vi "Z6_Beamline.panel.vi"(0 "object ref":refnum<vi>, 5 "error in (no error)":errorcluster) -> (19 "error out":errorcluster)   [LabVIEW 2014, in "Z6_Beamline.lvlib"]
doc: "By this VI a hardware switch can be monitored and switched. \n\nThe indicators \"FALSE\", \"TRUE\" and \"SWITCH STATE\" show the value of the Beckhoff-Tag: blue indicates bad tag status reference problems, darkgreen false and lightgreen true. If everything is working fine, \"FALSE\" and \"SWITCH STATE\" should show the same value, while \"TRUE\" has the opposite value. The caption of the sensors for \"FALSE\" and \"TRUE\" are taken out of the database. In case of only one or no sensor these GUI elements are not shown at all.\n\nThe oval button switches. It should be in the same state as the \"SWITCH STATE\" indicator. \n\n\"Delete Instance\" disconnects and removes the instance from the PCS.\n\n\nLicense Agreement for this software:\n\nCopyright (C)\nGesellschaft für Schwerionenforschung, GSI\nPlanckstr. 1\n64291 Darmstadt\nGermany\n\nContact: D.Beck@gsi.de \n\nThis program is free software; you can redistribute it and/or modify it under the terms of the GNU General Public License as published by the Free Software Foundation; either version 2 of the license, or (at your option) any later version.\n\nThis program is distributed in the hope that it will be useful, but WITHOUT ANYW ARRANTY; without even the implied warranty of MERCHANTABILITY or FITNESS FOR A PARTICULAR PURPOSE. See the GNU General License for more details (http://www.gnu.org).\n\nGesellschaft für Schwerionenforschung, GSI\nPlanckstr. 1, 64291 Darmstadt, Germany\nFor all questions and ideas contact: M.Richter@gsi.de, H.Brand@gsi.de or D.Beck@gsi.de.\nLast update: 18-DEC-2002"
uses:
  Z6_Beamline.lvlib
  PH_Common/Picture/PH_Picture.GUI Element 36x36.ctl
  PH_Common/Picture/PH_Picture.GUI Element 24x36.ctl
  PH_Common/Picture/PH_Picture.GUI Element.ctl
  Z6_Beamline.Switch Instances.ctl
  Z6_Beamline.Black Box Instances.ctl
  PH_SystemInformation/PH_SystemInformation.GUI Refs.ctl
  PH_BL-Master/PH_BL-Master.GUI Refs.ctl
  Z6_Beamline.Subsystem ok GUI Refs.ctl
  Z6_Beamline.GUI Refs.ctl
  PH_Common/PH_Common.lvlib
  PH_Switch/PH_Switch.lvlib
  PH_BlackBox/PH_BlackBox.lvlib
  PH_BL-Master/PH_BL-Master.lvlib
  PH_Class/PH_Class.lvlib
  PH_SystemInformation/PH_SystemInformation.lvlib
panel:
  in  "Z6 Black Box Instances":T1="Z6_ST_Attenuator_1_BB"
  in  "Z6 Switch Instances":T2="Shutter_Exp4"
  out "Exp 3":u32(colorbox)
  out "Exp 2":u32(colorbox)
  out "Exp 1":u32(colorbox)
  out "Emergency Off":u32(colorbox)
  in  "Remote Desktop Connection":bool
  out "PHELIX_Timing_Mode":enum32{"10 Hz", "0.5 Hz", "Shot"}(radio) caption="Modeselector"
  in  "PCS System Indicator":bool caption="PCS"
  in  "CoG":bool
  in  "Calibrator":bool
  in  "Image Statistician":bool
  in  "Z6 Main":bool
  out "Exp 4 (Z6)":u32(colorbox)
  in  "Tab Control":T3(tab)
  in  "PA_CH1_BB":T4 caption="CH"
  in  "ns_WP_RR_6PWpGUI":T5 caption="Waveplate ns Frontend"
  in  "YLF_WP_6PWpGUI":T5 caption="Waveplate YLF"
  in  "fs_WP_Exit_6PWpGUI":T5 caption="Waveplate fs Frontend"
  in  "Hop 3":bool
  out "Frontends ok":bool caption="ok"
  in  "MA_MM8_6PGUI":T6
  in  "MA_MM9_6PGUI":T6
  out "MA_VacuumControl::MA_VacuumControl_Z6 Telescope BL Prepressure":dbl=2000.0 caption="mbar" format="%#_2e"
  in  "BL-Z6-CH10":T4
  out "BL NT 2":u32(colorbox)
  in  "BL-Z6-CH9":T4
  in  "BL-Z6-Beamdump":bool=TRUE
  in  "Hop 4":bool
  in  "Z6_SHG_TIP-TILT_6PGUI":T6
  in  "Z6_SHG_ROT_6PGUI":T6
  out "MA_VacuumControl::MA_VacuumControl_Z6 Telescope BL":dbl=2000.0 caption="mbar" format="%#_2e"
  out "BL NT 3":u32(colorbox)
  in  "Z6_MM10_6PGUI":T6
  in  "Hop 1":bool
  out "Shutter_Exp4":bool=TRUE
  in  "\"D:\\PCS\\Remote Access\\Z6-Northtower.rdp\"":bool caption="OK Button"
  out "Northtower ok":bool caption="ok"
  in  "\"D:\\PCS\\Remote Access\\Z6-Southtower.rdp\"":bool caption="OK Button"
  out "Southtower ok":bool caption="ok"
  in  "Z6_ST_Attenuator_1_BB":bool=TRUE
  in  "Z6_ST_Attenuator_2_BB":T5 caption="BB 2"
  in  "Z6_green_Alignment_Powermeter":bool=TRUE
  in  "BL-Z6-CH11":T4
  in  "Z6_ST_WP_6PWpGUI":T5 caption="Waveplate"
  in  "Hop 5":bool
  in  "Z6_ST_NF_green_Cam":bool=TRUE caption="PA NF Exit Cam"
  in  "Z6_green_Powermeter":bool=TRUE
  out "BL ST 10":u32(colorbox)
  out "BL ST 9":u32(colorbox)
  out "BL ST 8":u32(colorbox)
  out "BL ST 7":u32(colorbox)
  in  "Z6_IR_Powermeter":bool=TRUE
  out "BL ST 6":u32(colorbox)
  in  "Z6_ST_NF_IR_Cam":bool=TRUE caption="PA FF Exit Cam"
  out "BL ST 5":u32(colorbox)
  out "BL ST 4":u32(colorbox)
  out "BL ST 3":u32(colorbox)
  out "BL ST 1":u32(colorbox)
  in  "Hop 2":bool
  out "BL ST 2":u32(colorbox)
  in  "Z6_MM11_6PGUI":T6
  in  "Z6_ST_Flip_Cam_BB":T6
  in  "Z6_ST_Flip_PD_BB":T6
  in  "\"D:\\PCS\\Remote Access\\Z6-Compressor.rdp\"":bool caption="OK Button"
  in  "Z6_ST_COS_Sensitivity_Switch_BB":bool=TRUE
  in  "Z6_ST_COS_WP_6PWpGUI":T5 caption="Waveplate"
  in  "Z6_ST_COS_Filt_1_BB":T5 caption="Filt 1"
  in  "Z6_ST_COS_Filt_2_BB":bool=TRUE
  in  "Z6_COS_Powermeter":bool=TRUE
  out "BL 100TW COS 6":u32(colorbox)
  out "BL 100TW COS 5":u32(colorbox)
  in  "Z6_Compressor-SSAC":bool=TRUE
  in  "Z6_COS_SSAC_Cam":bool=TRUE caption="PA NF Exit Cam"
  in  "Z6_COS_NF_ImageOperator":bool=TRUE
  in  "Z6_COS_NF_Cam":bool=TRUE caption="PA NF Exit Cam"
  in  "Z6_COS_FF_Cam":bool=TRUE caption="PA FF Exit Cam"
  in  "Hop 6":bool
  out "100TW COS ok":bool caption="ok"
  out "Ready for Shot":bool
  out "MainAmp enabled":u32(colorbox)
  out "Laser enabled":u32(colorbox)
  out "PreAmp enabled":u32(colorbox)
  in  "Minimize":bool
  in  "Delete":bool
  out "loop counter":i32
  # "Z6-CS"
  # "3.40"
  # "2"
  # "1"
  # "GREEN"
  # "IR"
  # "1"
  # "2"
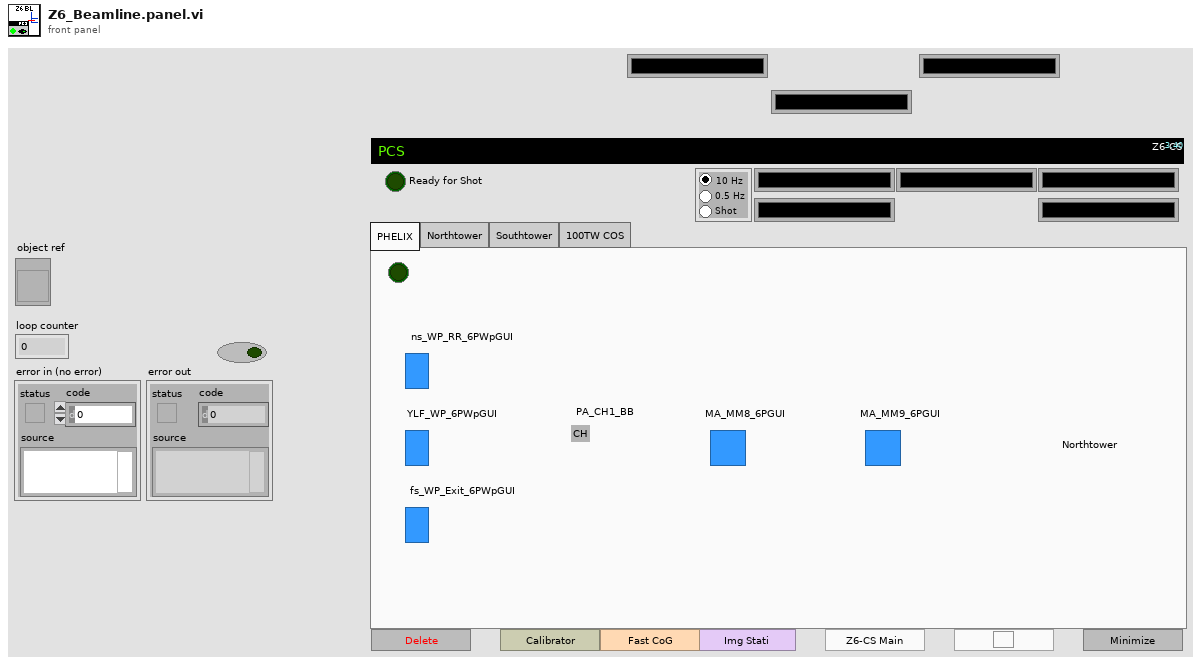
[diagram p1: front panel]
types:
  T1 = typedef "Z6_Beamline.lvlib/Z6_Beamline.Black Box Instances.ctl" = string
  T2 = typedef "Z6_Beamline.lvlib/Z6_Beamline.Switch Instances.ctl" = string
  T3 = enum32{"PHELIX", "Northtower", "Southtower", "100TW COS"}
  T4 = typedef "PH_Common.lvlib/PH_Picture.GUI Element.ctl" = picture
  T5 = typedef "PH_Common.lvlib/PH_Picture.GUI Element 24x36.ctl" = picture
  T6 = typedef "PH_Common.lvlib/PH_Picture.GUI Element 36x36.ctl" = picture
  T7 = typedef "Z6_Beamline.lvlib/Z6_Beamline.GUI Refs.ctl" = cluster{"BL NT":refnum<vi>[], "BL ST":refnum<vi>[], "BL 100 TW COS":refnum<vi>[], "Subs ok GUI Refs":T8}
  T8 = typedef "Z6_Beamline.lvlib/Z6_Beamline.Subsystem ok GUI Refs.ctl" = cluster{"Northtower ok":refnum<vi>, "Southtower ok":refnum<vi>, "Frontends ok":refnum<vi>, "100TW COS ok":refnum<vi>}
  T9 = typedef "PH_BL-Master.lvlib/PH_BL-Master.GUI Refs.ctl" = cluster{"Vac GUI Refs":refnum<vi>[], "O2 GUI Refs":refnum<vi>[], "Ready for Shot":refnum<vi>, "Boolean Condition Service Subscriber GUI Refs":refnum<vi>[], "Vision ID on same Node":string, "Picture Condition Service Subscriber GUI Refs":refnum<vi>[], "6P 4Q GUI Refs":refnum<vi>[], "Ref Switch GUI Instances":refnum<vi>, "Ref 6P Switch Instances":refnum<vi>, "Ref BB Instances":refnum<vi>, "Ref Switch Instances":refnum<vi>, "Ref Switch and 6P State Instances":refnum<vi>, "Boolean Status Service Subscriber GUI Refs":refnum<vi>[], "Picture Status Service Subscriber GUI Refs":refnum<vi>[], "Force Sensor Instances":refnum<vi>, "GUI Ref Delete":refnum<vi>}
  T10 = typedef "PH_SystemInformation.lvlib/PH_SystemInformation.GUI Refs.ctl" = cluster{"Laser":refnum<vi>, "PreAmp":refnum<vi>, "MainAmp":refnum<vi>, "Emergency Off":refnum<vi>, "Exp 1":refnum<vi>, "Exp 2":refnum<vi>, "Exp 3":refnum<vi>, "Exp 4":refnum<vi>, "Timing Mode GUI Ref":refnum<vi>}
  T11 = enum16{"PCS", "Laser", "Vision", "PP", "Special", "Beckhoff"}
  T12 = enum16{"None", "PCS Main", "Z6 Main", "PCS Beamline", "Z6 Beamline", "Image Statistician", "Powermeter Statistician", "SHS Anal Statistician", "Image Center of Gravity", "Image Calibrator", "SHS Analysis Calibrator", "Cam List", "Powermeterlist", "6P List", "BB List", "Switch List", "Sequence Watch"}
  T13 = typedef "PH_BL-Master.lvlib/PH_BL-Master.i attribute.ctl" = cluster{"Remote controlled":bool, "Boolean Condition Service Subscriber":refnum<vi>[], "Picture Condition Service Subscriber":refnum<vi>[], "R2S":cluster{"GUI Ref":refnum<vi>, "State":bool}, "Vacua":cluster{"GUI Ref":refnum<vi>, "Limit":dbl, "Curr Value":dbl, "in range":bool}[], "O2 Inspection":cluster{"GUI Ref":refnum<vi>, "Concentration":dbl, "State":T14}[], "Boolean Status Service Subscriber":cluster{"GUI Ref":refnum<vi>, "Status":T14, "no Link?":bool, "Status Subscriber Class":T15}[], "Picture Status Service Subscriber":cluster{"GUI Ref":refnum<vi>, "Status":T14, "no Link?":bool, "Status Subscriber Class":T15}[], "6P 4Q Service Subscriber":cluster{"GUI Ref":refnum<vi>, "Selector":T16, "no Link?":bool}[], "Index of latest 6P 4Q changing Instance":i32, "Index of latest Picture Status changing Instance":i32, "Index of latest Boolean Status changing Instance":i32, "Vision ID on same Node":string, "Start Phase over?":bool, "GUI Ref Delete":refnum<vi>}
  T14 = typedef "PH_StatusHandler.lvlib/PH_StatusHandler.Status.ctl" = i16
  T15 = typedef "PH_BL-Master.lvlib/PH_BL-Master.Status Subscriber Class.ctl" = enum16{"unknown", "Switch", "BB", "6P Switch", "Switch GUI", "Switch and 6P State", "Force Sensor"}
  T16 = typedef "PH_4_Pos_Selector.lvlib/PH_4_Pos_Selector.Position Selector.ctl" = u16
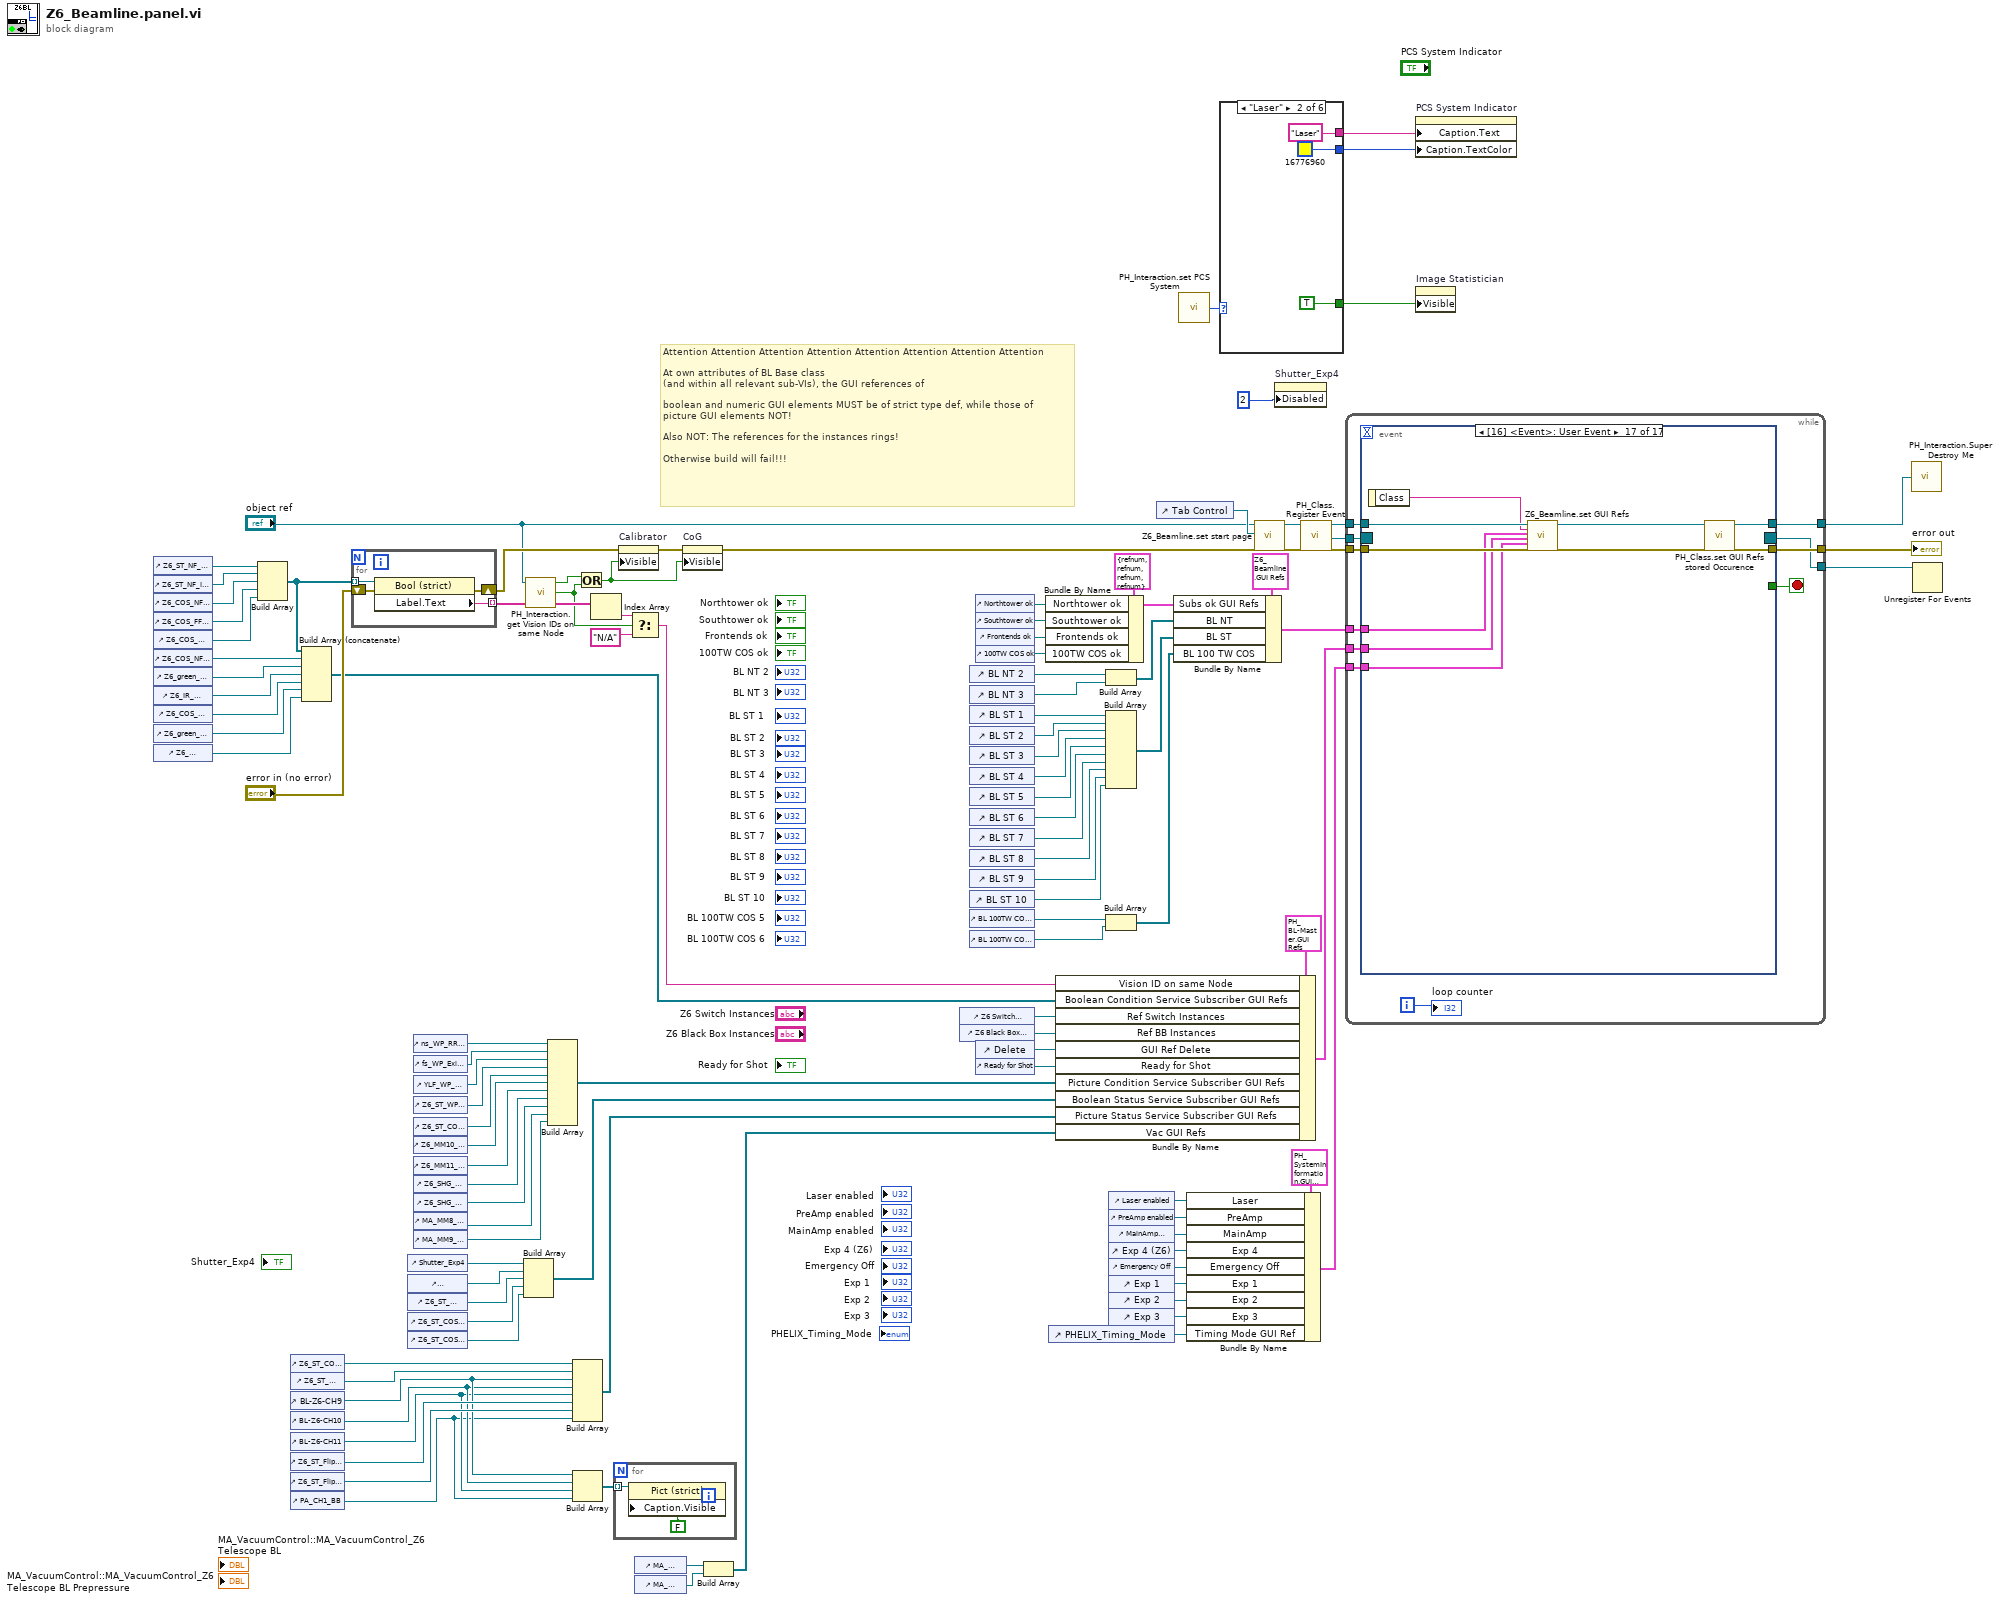
[diagram p0: block diagram]
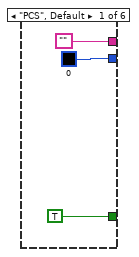
[diagram p2: hidden frame]
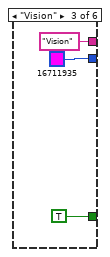
[diagram p3: hidden frame]
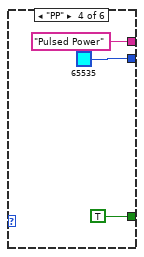
[diagram p4: hidden frame]
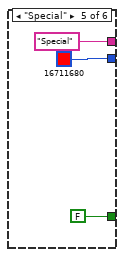
[diagram p5: hidden frame]
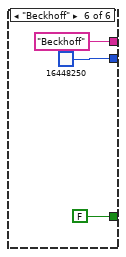
[diagram p6: hidden frame]
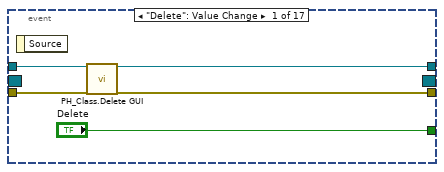
[diagram p7: hidden frame]
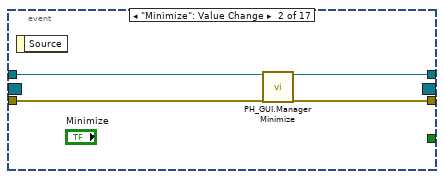
[diagram p8: hidden frame]
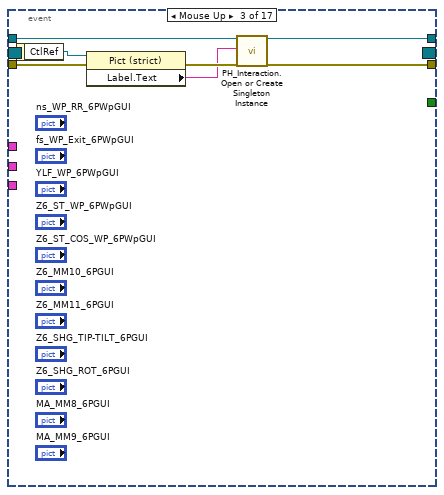
[diagram p9: hidden frame]
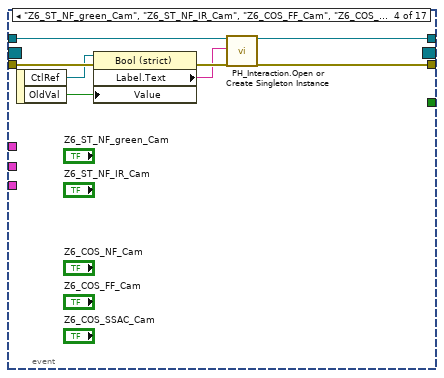
[diagram p10: hidden frame]
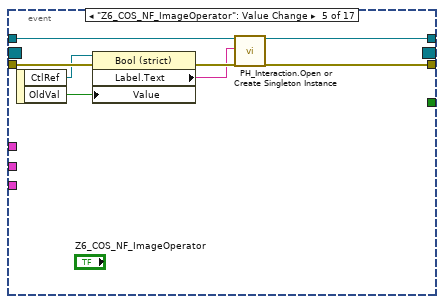
[diagram p11: hidden frame]
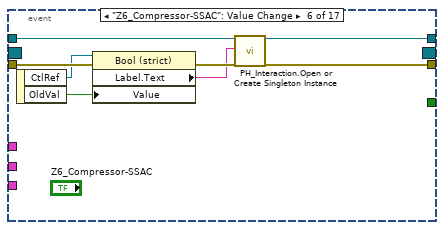
[diagram p12: hidden frame]
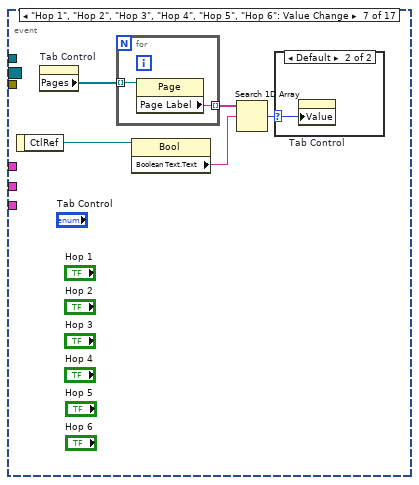
[diagram p13: hidden frame]
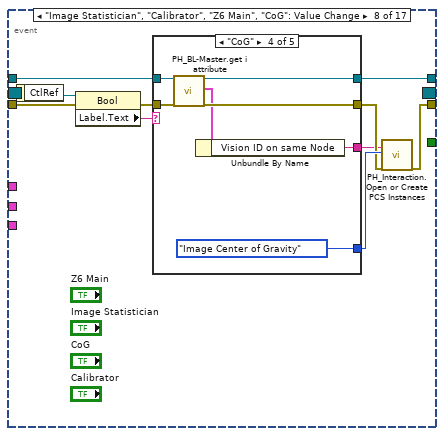
[diagram p15: hidden frame]
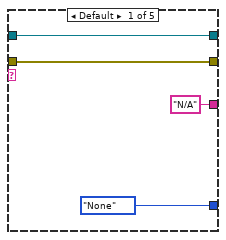
[diagram p16: hidden frame]
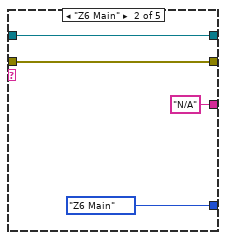
[diagram p17: hidden frame]
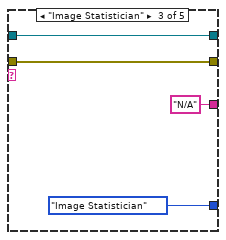
[diagram p18: hidden frame]
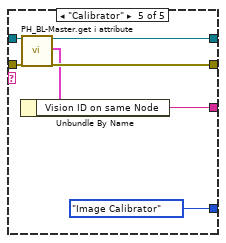
[diagram p19: hidden frame]
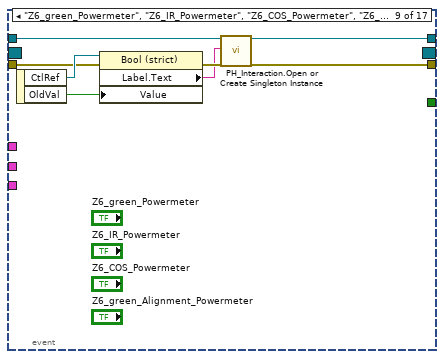
[diagram p20: hidden frame]
diagram:
  # "Attention Attention Attention Attention Attention Attention Attention Attention\n\nAt own attributes of BL Base class \n(and within all relevant sub-VIs), the GUI references of\n\nboolean and numeric GUI elements MUST be of strict type def, while those of\npicture GUI elements NOT!\n\nAlso NOT: The references for the instances rings!\n\nOtherwise build will fail!!!"
  n1 = control-ref of="Z6_ST_NF_green_Cam"() -> (w48:refnum<vi>)
  n2 = control-ref of="Z6_ST_NF_IR_Cam"() -> (w47:refnum<vi>)
  n3 = control-ref of="Z6_COS_NF_Cam"() -> (w46:refnum<vi>)
  n4 = control-ref of="Z6_COS_FF_Cam"() -> (w45:refnum<vi>)
  n5 = control-ref of="Z6_COS_SSAC_Cam"() -> (w44:refnum<vi>)
  n6 = control-ref of="Z6_COS_NF_ImageOperator"() -> (w67:refnum<vi>)
  n7 = control-ref of="Z6_green_Powermeter"() -> (w64:refnum<vi>)
  n8 = control-ref of="Z6_IR_Powermeter"() -> (w63:refnum<vi>)
  n9 = control-ref of="Z6_COS_Powermeter"() -> (w62:refnum<vi>)
  n10 = control-ref of="Z6_green_Alignment_Powermeter"() -> (w61:refnum<vi>)
  n11 = control-ref of="Z6_Compressor-SSAC"() -> (w60:refnum<vi>)
  n12 = Build Array(w48, w47, w46, w45, w44) -> (w43:refnum<vi>[])
  n13 = control-ref of="Z6_ST_COS_Filt_1_BB"() -> (w88:refnum<vi>)
  n14 = control-ref of="Z6_ST_Attenuator_2_BB"() -> (w87:refnum<vi>)
  n15 = control-ref of="BL-Z6-CH9"() -> (w75:refnum<vi>)
  n16 = control-ref of="BL-Z6-CH10"() -> (w74:refnum<vi>)
  n17 = control-ref of="BL-Z6-CH11"() -> (w73:refnum<vi>)
  n18 = control-ref of="Z6_ST_Flip_Cam_BB"() -> (w79:refnum<vi>)
  n19 = control-ref of="Z6_ST_Flip_PD_BB"() -> (w78:refnum<vi>)
  n20 = control-ref of="PA_CH1_BB"() -> (w56:refnum<vi>)
  n21 = Build Array (concatenate)(w43, w67, w64, w63, w62, w61, w60) -> (w2:refnum<vi>[])
  n22 = for {
    shift-right: [w115] -> w22
    shift-left: "error in (no error)" -> [w116]
    tunnel: [w114] -> w51 mode=indexing
    tunnel: w43 -> [w113] mode=indexing
    n23 = property class="Bool (strict)"(reference=w113, error in=w116) -> (error out=w115:errorcluster, "Label.Text"=w114:string)  [unwired: 1 out]
  }
  n24 = control-ref of="Shutter_Exp4"() -> (w66:refnum<vi>)
  n25 = control-ref of="BL-Z6-Beamdump"() -> (w65:refnum<vi>)
  n26 = control-ref of="Z6_ST_Attenuator_1_BB"() -> (w59:refnum<vi>)
  n27 = control-ref of="Z6_ST_COS_Sensitivity_Switch_BB"() -> (w58:refnum<vi>)
  n28 = control-ref of="Z6_ST_COS_Filt_2_BB"() -> (w57:refnum<vi>)
  n29 = control-ref of="ns_WP_RR_6PWpGUI"() -> (w86:refnum<vi>)
  n30 = control-ref of="fs_WP_Exit_6PWpGUI"() -> (w85:refnum<vi>)
  n31 = control-ref of="YLF_WP_6PWpGUI"() -> (w84:refnum<vi>)
  n32 = control-ref of="Z6_ST_WP_6PWpGUI"() -> (w83:refnum<vi>)
  n33 = control-ref of="Z6_ST_COS_WP_6PWpGUI"() -> (w82:refnum<vi>)
  n34 = control-ref of="Z6_MM10_6PGUI"() -> (w81:refnum<vi>)
  n35 = control-ref of="Z6_MM11_6PGUI"() -> (w80:refnum<vi>)
  n36 = control-ref of="Z6_SHG_ROT_6PGUI"() -> (w77:refnum<vi>)
  n37 = control-ref of="Z6_SHG_TIP-TILT_6PGUI"() -> (w76:refnum<vi>)
  n38 = control-ref of="MA_MM8_6PGUI"() -> (w39:refnum<vi>)
  n39 = control-ref of="MA_MM9_6PGUI"() -> (w38:refnum<vi>)
  n40 = Build Array(w66, w65, w59, w58, w57) -> (w25:refnum<vi>[])
  n41 = call "PH_Interaction.get Vision IDs on same Node.vi"("Cam Instances"=w51, "i ref in"="object ref") -> ("Vision System IDs"=w42:string[], "Vision Sytem IDs found"=w40:bool, "Cams instanciated on own system"=w41:bool)  [unwired: 1 in]
  n42 = Build Array(w86, w85, w84, w83, w82, w81, w80, w77, w76, w39, w38) -> (w26:refnum<vi>[])
  n43 = Build Array(w88, w87, w75, w74, w73, w79, w78, w56) -> (w24:refnum<vi>[])
  n44 = Build Array(w75, w74, w73, w56) -> (w72:refnum<vi>[])
  n45 = Or(x=w41, y=w40) -> (x .or. y?=w21:bool)
  n46 = Index Array(array=w42) -> (element=w50:string)  [unwired: 1 in]
  n47 = for {
    tunnel: w72 -> [w118] mode=indexing
    n48 = property class="Pict (strict)"(reference=w118, "Caption.Visible"=FALSE) -> ()  [unwired: 1 in, 2 out]
  }
  n49 = property on="Calibrator" class="Bool"(error in=w22, "Visible"=w21) -> (error out=w23:errorcluster)  [unwired: 1 in, 1 out]
  n50 = Select(t=w50, s=w40, f="N/A") -> (s? t:f=w3:string)
  n51 = control-ref of="MA_VacuumControl::MA_VacuumControl_Z6 Telescope BL"() -> (w107:refnum<vi>)
  n52 = control-ref of="MA_VacuumControl::MA_VacuumControl_Z6 Telescope BL Prepressure"() -> (w37:refnum<vi>)
  n53 = property on="CoG" class="Bool"(error in=w23, "Visible"=w21) -> (error out=w18:errorcluster)  [unwired: 1 in, 1 out]
  n54 = Build Array(w107, w37) -> (w1:refnum<vi>[])
  n55 = control-ref of="Z6 Switch Instances"() -> (w29:refnum<vi>)
  n56 = control-ref of="Z6 Black Box Instances"() -> (w28:refnum<vi>)
  n57 = control-ref of="BL NT 2"() -> (w111:refnum<vi>)
  n58 = control-ref of="BL NT 3"() -> (w110:refnum<vi>)
  n59 = control-ref of="BL ST 1"() -> (w106:refnum<vi>)
  n60 = control-ref of="BL ST 2"() -> (w105:refnum<vi>)
  n61 = control-ref of="BL ST 3"() -> (w96:refnum<vi>)
  n62 = control-ref of="BL ST 4"() -> (w95:refnum<vi>)
  n63 = control-ref of="BL ST 5"() -> (w94:refnum<vi>)
  n64 = control-ref of="BL ST 6"() -> (w93:refnum<vi>)
  n65 = control-ref of="BL ST 7"() -> (w92:refnum<vi>)
  n66 = control-ref of="BL ST 8"() -> (w91:refnum<vi>)
  n67 = control-ref of="BL ST 9"() -> (w90:refnum<vi>)
  n68 = control-ref of="BL ST 10"() -> (w89:refnum<vi>)
  n69 = control-ref of="BL 100TW COS 5"() -> (w103:refnum<vi>)
  n70 = control-ref of="BL 100TW COS 6"() -> (w102:refnum<vi>)
  n71 = control-ref of="Northtower ok"() -> (w11:refnum<vi>)
  n72 = control-ref of="Southtower ok"() -> (w10:refnum<vi>)
  n73 = control-ref of="Frontends ok"() -> (w9:refnum<vi>)
  n74 = control-ref of="100TW COS ok"() -> (w8:refnum<vi>)
  n75 = control-ref of="Delete"() -> (w6:refnum<vi>)
  n76 = control-ref of="Ready for Shot"() -> (w27:refnum<vi>)
  n77 = Bundle By Name(cluster=T8 {"Northtower ok"=refnum, "Southtower ok"=refnum, "Frontends ok"=refnum, "100TW COS ok"=refnum} ("Subs ok GUI Refs"), "Northtower ok"=w11, "Southtower ok"=w10, "Frontends ok"=w9, "100TW COS ok"=w8) -> (w12:T8)
  n78 = control-ref of="PHELIX_Timing_Mode"() -> (w36:refnum<vi>)
  n79 = Bundle By Name(cluster=T9 {"Vac GUI Refs"=[], "O2 GUI Refs"=[], "Ready for Shot"=refnum, "Boolean Condition Service Subscriber GUI Refs"=[], "Vision ID on same Node"="", "Picture Condition Service Subscriber GUI Refs"=[], "6P 4Q GUI Refs"=[], "Ref Switch GUI Instances"=refnum, "Ref 6P Switch Instances"=refnum, "Ref BB Instances"=refnum, "Ref Switch Instances"=refnum, "Ref Switch and 6P State Instances"=refnum, "Boolean Status Service Subscriber GUI Refs"=[], "Picture Status Service Subscriber GUI Refs"=[], "Force Sensor Instances"=refnum, "GUI Ref Delete"=refnum} ("PH_BL_Master GUI Refs"), "Vision ID on same Node"=w3, "Boolean Condition Service Subscriber GUI Refs"=w2, "Ref Switch Instances"=w29, "Ref BB Instances"=w28, "GUI Ref Delete"=w6, "Ready for Shot"=w27, "Picture Condition Service Subscriber GUI Refs"=w26, "Boolean Status Service Subscriber GUI Refs"=w25, "Picture Status Service Subscriber GUI Refs"=w24, "Vac GUI Refs"=w1) -> (w4:T9)
  n80 = Build Array(w111, w110) -> (w16:refnum<vi>[])
  n81 = Build Array(w106, w105, w96, w95, w94, w93, w92, w91, w90, w89) -> (w15:refnum<vi>[])
  n82 = Build Array(w103, w102) -> (w14:refnum<vi>[])
  n83 = control-ref of="Laser enabled"() -> (w97:refnum<vi>)
  n84 = control-ref of="PreAmp enabled"() -> (w98:refnum<vi>)
  n85 = control-ref of="MainAmp enabled"() -> (w99:refnum<vi>)
  n86 = control-ref of="Exp 4 (Z6)"() -> (w100:refnum<vi>)
  n87 = control-ref of="Emergency Off"() -> (w71:refnum<vi>)
  n88 = control-ref of="Exp 1"() -> (w70:refnum<vi>)
  n89 = control-ref of="Exp 2"() -> (w69:refnum<vi>)
  n90 = control-ref of="Exp 3"() -> (w68:refnum<vi>)
  n91 = control-ref of="Tab Control"() -> (w104:refnum<vi>)
  n92 = Bundle By Name(cluster=T7 {"BL NT"=[], "BL ST"=[], "BL 100 TW COS"=[], "Subs ok GUI Refs"={"Northtower ok"=refnum, "Southtower ok"=refnum, "Frontends ok"=refnum, "100TW COS ok"=refnum}} ("Z6 Beamline GUI Refs"), "Subs ok GUI Refs"=w12, "BL NT"=w16, "BL ST"=w15, "BL 100 TW COS"=w14) -> (w17:T7)
  n93 = call "PH_Interaction.set PCS System.vi"() -> ("Enum"=w55:T11)  [unwired: 1 in]
  n94 = Bundle By Name(cluster=T10 {"Laser"=refnum, "PreAmp"=refnum, "MainAmp"=refnum, "Emergency Off"=refnum, "Exp 1"=refnum, "Exp 2"=refnum, "Exp 3"=refnum, "Exp 4"=refnum, "Timing Mode GUI Ref"=refnum} ("System Information GUI Refs"), "Laser"=w97, "PreAmp"=w98, "MainAmp"=w99, "Exp 4"=w100, "Emergency Off"=w71, "Exp 1"=w70, "Exp 2"=w69, "Exp 3"=w68, "Timing Mode GUI Ref"=w36) -> (w5:T10)
  n95 = case shown="\"Laser\"" w55 {
    tunnel: ["" "Laser" "Vision" "Pulsed Power" "Special" "Beckhoff"] -> w54
    tunnel: [TRUE TRUE TRUE TRUE FALSE FALSE] -> w52
    tunnel: [u32 0 ("Color Box") u32 16776960 ("Color Box") u32 16711935 ("Color Box") u32 65535 ("Color Box") u32 16711680 ("Color Box") u32 16448250 ("Color Box")] -> w53
    frame "PCS", Default {
    }
    frame "Laser" {
    }
    frame "Vision" {
    }
    frame "PP" {
    }
    frame "Special" {
    }
    frame "Beckhoff" {
    }
  }
  n96 = call "Z6_Beamline.set start page.vi"("i ref in"="object ref", "Tab Control"=w104, "error in (no error)"=w18) -> ("i ref out"=w20:refnum<vi>)  [unwired: 15 in, 1 out]
  n97 = property on="Shutter_Exp4" class="Bool (strict)"("Disabled"=u8 2) -> ()  [unwired: 2 in, 2 out]
  n98 = call "PH_Class.Register Event.vi"("i ref in"=w20, "error in (no error)"=w18) -> ("i ref out"=w34:refnum<vi>, "Event Registration Refnum"=w33:refnum<event-registration>, "error out"=w35:errorcluster)  [unwired: 15 in]
  n99 = while {
    tunnel: w34 -> [w144]
    tunnel: [w143] -> w109
    tunnel: w35 -> [w146]
    tunnel: [w145] -> w108
    tunnel: w33 -> [w141]
    tunnel: [w140] -> w32
    tunnel: w17 -> [w139]
    tunnel: w5 -> [w138]
    tunnel: w4 -> [w137]
    i -> [w147]
    stop <- w142 stop-if-true
    n100 = event shown="[16] <Event>: User Event" {
      selector: w141 -> [_ _ _ _ _ _ _ _ _ _ _ _ _ _ _ _ _]
      dyn-events: [_ _ _ _ _ _ _ _ _ _ _ _ _ _ _ _ _] -> w140
      timeout: _ -> [_ _ _ _ _ _ _ _ _ _ _ _ _ _ _ _ _]
      tunnel: w144 -> [w152 w156 w159 w169 w175 w183 _ w198 w237 w247 w270 w283 w291 w298 w305 w319 w335]
      tunnel: w146 -> [w150 w155 w162 w168 w177 w185 _ w205 w238 w249 w268 w282 w289 w297 w316 w320 w337]
      tunnel: [w148 w154 w160 w170 w178 w186 _ w204 w233 w243 w264 w286 w294 w301 w306 w318 w339] -> w145
      tunnel: [w149 w153 w161 w171 w179 w187 _ w197 w234 w246 w262 w285 w293 w300 w305 w319 w338] -> w143
      tunnel: ["Delete" _ _ _ _ _ _ _ _ _ _ _ _ _ _ _ _] -> w142
      tunnel: w139 -> [_ _ _ _ _ _ _ _ _ _ _ _ _ _ _ _ w332]
      tunnel: w138 -> [_ _ _ _ _ _ _ _ _ _ _ _ _ _ _ _ w330]
      tunnel: w137 -> [_ _ _ _ _ _ _ _ _ _ _ _ _ _ _ _ w331]
      event "Delete": Value Change {
        n101 = event-data() -> ()  [unwired: 1 in, 1 out]
        n102 = call "PH_Class.Delete GUI.vi"("VI in"=w152, "error in (no error)"=w150) -> ("VI out"=w149:refnum<vi>, "error out"=w148:errorcluster)  [unwired: 16 in]
      }
      event "Minimize": Value Change {
        n103 = event-data() -> ()  [unwired: 1 in, 1 out]
        n104 = call "PH_GUI.Manager Minimize.vi"("i ref in"=w156, "error in"=w155) -> ("i ref out"=w153:refnum<vi>, "error out"=w154:errorcluster)  [unwired: 16 in]
      }
      event Mouse Up {
        n105 = event-data() -> ("CtlRef"=w163:refnum<vi>)  [unwired: 1 in]
        n106 = property class="Pict (strict)"(reference=w163, error in=w162) -> (error out=w158:errorcluster, "Label.Text"=w157:string)  [unwired: 1 out]
        n107 = call "PH_Interaction.Open or Create Singleton Instance.vi"("i ref in"=w159, "Instance to create or to open"=w157, "error IO"=w158) -> ("i ref out"=w161:refnum<vi>, "error out"=w160:errorcluster)  [unwired: 15 in]
      }
      event "Z6_ST_NF_green_Cam", "Z6_ST_NF_IR_Cam", "Z6_COS_FF_Cam", "Z6_COS_NF_Cam", "Z6_COS_SSAC_Cam": Value Change {
        n108 = event-data() -> ("CtlRef"=w167:refnum<vi>, "OldVal"=w164:bool)  [unwired: 1 in]
        n109 = property class="Bool (strict)"(reference=w167, error in=w168, "Value"=w164) -> (error out=w166:errorcluster, "Label.Text"=w165:string)  [unwired: 1 out]
        n110 = call "PH_Interaction.Open or Create Singleton Instance.vi"("i ref in"=w169, "Instance to create or to open"=w165, "error IO"=w166) -> ("i ref out"=w171:refnum<vi>, "error out"=w170:errorcluster)  [unwired: 15 in]
      }
      event "Z6_COS_NF_ImageOperator": Value Change {
        n111 = event-data() -> ("CtlRef"=w173:refnum<vi>, "OldVal"=w172:bool)  [unwired: 1 in]
        n112 = property class="Bool (strict)"(reference=w173, error in=w177, "Value"=w172) -> (error out=w176:errorcluster, "Label.Text"=w174:string)  [unwired: 1 out]
        n113 = call "PH_Interaction.Open or Create Singleton Instance.vi"("i ref in"=w175, "Instance to create or to open"=w174, "error IO"=w176) -> ("i ref out"=w179:refnum<vi>, "error out"=w178:errorcluster)  [unwired: 15 in]
      }
      event "Z6_Compressor-SSAC": Value Change {
        n114 = event-data() -> ("CtlRef"=w181:refnum<vi>, "OldVal"=w180:bool)  [unwired: 1 in]
        n115 = property class="Bool (strict)"(reference=w181, error in=w185, "Value"=w180) -> (error out=w184:errorcluster, "Label.Text"=w182:string)  [unwired: 1 out]
        n116 = call "PH_Interaction.Open or Create Singleton Instance.vi"("i ref in"=w183, "Instance to create or to open"=w182, "error IO"=w184) -> ("i ref out"=w187:refnum<vi>, "error out"=w186:errorcluster)  [unwired: 15 in]
      }
      event "Hop 1", "Hop 2", "Hop 3", "Hop 4", "Hop 5", "Hop 6": Value Change {
        n117 = event-data() -> ("CtlRef"=w192:refnum<vi>)  [unwired: 1 in]
        n118 = property on="Tab Control" class="TabCtl (strict)"() -> ("Pages"=w188:refnum<vi>[])  [unwired: 2 in, 2 out]
        n119 = for {
          tunnel: [w195] -> w191 mode=indexing
          tunnel: w188 -> [w194] mode=indexing
          n120 = property class="Page"(reference=w194) -> ("Page Label"=w195:string)  [unwired: 1 in, 2 out]
        }
        n121 = property class="Bool"(reference=w192) -> ("Boolean Text.Text"=w190:string)  [unwired: 1 in, 2 out]
        n122 = Search 1D Array(1D array=w191, element=w190) -> (index of element=w189:i32)  [unwired: 1 in]
        n123 = case shown="Default" w189 {
          selector: w189 -> [_ w193]
          frame -1 {
          }
          frame Default {
            n124 = property on="Tab Control" class="TabCtl (strict)"("Value"=w193) -> ()  [unwired: 2 in, 2 out]
          }
        }
      }
      event "Image Statistician", "Calibrator", "Z6 Main", "CoG": Value Change {
        n125 = event-data() -> ("CtlRef"=w203:refnum<vi>)  [unwired: 1 in]
        n126 = property class="Bool"(reference=w203, error in=w205) -> (error out=w200:errorcluster, "Label.Text"=w201:string)  [unwired: 1 out]
        n127 = case shown="\"CoG\"" w201 {
          tunnel: [T12."None" ("Instance to create or open") T12."Z6 Main" ("Instance to create or open") T12."Image Statistician" ("Instance to create or open") T12."Image Center of Gravity" ("Instance to create or open") T12."Image Calibrator" ("Instance to create or open")] -> w202
          tunnel: w200 -> [w207 w211 w215 w222 w230]
          tunnel: [w207 w211 w215 w220 w229] -> w199
          tunnel: w198 -> [w208 w212 w216 w223 w228]
          tunnel: [w208 w212 w216 w221 w227] -> w197
          tunnel: ["N/A" ("Vision ID on same Node") "N/A" ("Vision ID on same Node") "N/A" ("Vision ID on same Node") w218 w225] -> w196
          frame Default {
          }
          frame "Z6 Main" {
          }
          frame "Image Statistician" {
          }
          frame "CoG" {
            n128 = call "PH_BL-Master.get i attribute.vi"("i ref in"=w223, "error in (no error)"=w222) -> ("i ref out"=w221:refnum<vi>, "i attribute"=w219:T13, "error out"=w220:errorcluster)  [unwired: 15 in]
            n129 = Unbundle By Name(w219) -> ("Vision ID on same Node"=w218:string)
          }
          frame "Calibrator" {
            n130 = call "PH_BL-Master.get i attribute.vi"("i ref in"=w228, "error in (no error)"=w230) -> ("i ref out"=w227:refnum<vi>, "i attribute"=w226:T13, "error out"=w229:errorcluster)  [unwired: 15 in]
            n131 = Unbundle By Name(w226) -> ("Vision ID on same Node"=w225:string)
          }
        }
        n132 = call "PH_Interaction.Open or Create PCS Instances.vi"("System ID (N/A)"=w196, "Instance to create or open"=w202, "error IO"=w199) -> ("error out"=w204:errorcluster)  [unwired: 16 in]
      }
      event "Z6_green_Powermeter", "Z6_IR_Powermeter", "Z6_COS_Powermeter", "Z6_green_Alignment_Powermeter": Value Change {
        n133 = event-data() -> ("CtlRef"=w239:refnum<vi>, "OldVal"=w232:bool)  [unwired: 1 in]
        n134 = property class="Bool (strict)"(reference=w239, error in=w238, "Value"=w232) -> (error out=w236:errorcluster, "Label.Text"=w235:string)  [unwired: 1 out]
        n135 = call "PH_Interaction.Open or Create Singleton Instance.vi"("i ref in"=w237, "Instance to create or to open"=w235, "error IO"=w236) -> ("i ref out"=w234:refnum<vi>, "error out"=w233:errorcluster)  [unwired: 15 in]
      }
      event "BL-Z6-Beamdump": Value Change {
        n136 = event-data() -> ("CtlRef"=w241:refnum<vi>, "OldVal"=w240:bool)  [unwired: 1 in]
        n137 = property class="Bool (strict)"(reference=w241, error in=w249) -> (error out=w248:errorcluster, "Label.Text"=w245:string, "Value"=w244:bool)  [unwired: 1 out]
        n138 = case shown="False" w244 {
          tunnel: w247 -> [w254 w259]
          tunnel: [w253 w256] -> w246
          tunnel: w248 -> [w252 w258]
          tunnel: [w251 w257] -> w242
          tunnel: w245 -> [w250 w255]
          frame False {
            n139 = call "PH_Switch.evt false.vi"("i ref in"=w254, "Instance"=w250, "error in (no error)"=w252) -> ("i ref out"=w253:refnum<vi>, "error out"=w251:errorcluster)  [unwired: 15 in]
          }
          frame True {
            n140 = call "PH_Switch.evt true.vi"("i ref in"=w259, "Instance"=w255, "error in (no error)"=w258) -> ("i ref out"=w256:refnum<vi>, "error out"=w257:errorcluster)  [unwired: 15 in]
          }
        }
        n141 = property class="Bool (strict)"(reference=w241, error in=w242, "Value"=w240) -> (error out=w243:errorcluster)  [unwired: 1 out]
      }
      event Mouse Down {
        n142 = event-data() -> ("CtlRef"=w269:refnum<vi>)  [unwired: 1 in]
        n143 = property class="Pict (strict)"(reference=w269, error in=w268) -> (error out=w267:errorcluster, "Label.Text"=w260:string)  [unwired: 1 out]
        n144 = call "PH_BL-Master.get Picture Status Service Subscriber Status by Name.vi"("i ref in"=w270, "Picture Status Subscriber Instance"=w260, "error in (no error)"=w267) -> ("i ref out"=w263:refnum<vi>, "on/true/in?"=w261:bool, "error out"=w265:errorcluster)  [unwired: 7 in, 7 out]
        n145 = Not(x=w261) -> (.not. x?=w266:bool)
        n146 = case shown="False" w266 {
          tunnel: w263 -> [w275 w280]
          tunnel: [w274 w277] -> w262
          tunnel: w265 -> [w273 w279]
          tunnel: [w272 w278] -> w264
          tunnel: w260 -> [w271 w276]
          frame False {
            n147 = call "PH_Switch.evt false.vi"("i ref in"=w275, "Instance"=w271, "error in (no error)"=w273) -> ("i ref out"=w274:refnum<vi>, "error out"=w272:errorcluster)  [unwired: 15 in]
          }
          frame True {
            n148 = call "PH_Switch.evt true.vi"("i ref in"=w280, "Instance"=w276, "error in (no error)"=w279) -> ("i ref out"=w277:refnum<vi>, "error out"=w278:errorcluster)  [unwired: 15 in]
          }
        }
      }
      event Mouse Up {
        n149 = event-data() -> ("CtlRef"=w281:refnum<vi>)  [unwired: 1 in]
        n150 = property class="Pict (strict)"(reference=w281, error in=w282) -> (error out=w284:errorcluster, "Label.Text"=w287:string)  [unwired: 1 out]
        n151 = call "PH_BlackBox.evt start move.vi"("i ref in"=w283, "Instance"=w287, "error in (no error)"=w284) -> ("i ref out"=w285:refnum<vi>, "error out"=w286:errorcluster)  [unwired: 15 in]
      }
      event "Z6_ST_COS_Filt_2_BB", "Z6_ST_Attenuator_1_BB", "Z6_ST_COS_Sensitivity_Switch_BB": Value Change {
        n152 = event-data() -> ("CtlRef"=w288:refnum<vi>, "OldVal"=w290:bool)  [unwired: 1 in]
        n153 = property class="Bool (strict)"(reference=w288, error in=w289, "Value"=w290) -> (error out=w292:errorcluster, "Label.Text"=w295:string)  [unwired: 1 out]
        n154 = call "PH_BlackBox.evt start move.vi"("i ref in"=w291, "Instance"=w295, "error in (no error)"=w292) -> ("i ref out"=w293:refnum<vi>, "error out"=w294:errorcluster)  [unwired: 15 in]
      }
      event Mouse Down {
        n155 = event-data() -> ("CtlRef"=w296:refnum<vi>)  [unwired: 1 in]
        n156 = property class="Pict (strict)"(reference=w296, error in=w297) -> (error out=w299:errorcluster, "Label.Text"=w302:string)  [unwired: 1 out]
        n157 = call "PH_BlackBox.evt start move.vi"("i ref in"=w298, "Instance"=w302, "error in (no error)"=w299) -> ("i ref out"=w300:refnum<vi>, "error out"=w301:errorcluster)  [unwired: 15 in]
      }
      event "\"D:\\PCS\\Remote Access\\Z6-Northtower.rdp\"", "\"D:\\PCS\\Remote Access\\Z6-Southtower.rdp\"", "\"D:\\PCS\\Remote Access\\Z6-Compressor.rdp\"": Value Change {
        n158 = event-data() -> ("CtlRef"=w317:refnum<vi>)  [unwired: 1 in]
        n159 = property class="Bool"(reference=w317, error in=w316) -> (error out=w303:errorcluster, "Label.Text"=w304:string)  [unwired: 1 out]
        n160 = Match Pattern(string=w304, regular expression=" 2") -> (before substring=w307:string, offset past match=w311:i32)  [unwired: 1 in, 2 out]
        n161 = Equal?(x=w311, y=-1) -> (x = y?=w309:bool)
        n162 = Select(t=w304, s=w309, f=w307) -> (s? t:f=w308:string)
        n163 = Concatenate Strings("mstsc " ("command line"), w308) -> (w314:string)
        n164 = call <vilib>:"System Exec.vi"("wait until completion? (T)"=FALSE, "error in (no error)"=w303, "command line"=w314) -> ("error out"=w306:errorcluster)  [unwired: 5 in, 3 out]
      }
      event "Remote Desktop Connection": Value Change {
        n165 = event-data() -> ()  [unwired: 1 in, 1 out]
        n166 = call "PH_Connection.select PCS Node.vi"("error in"=w320) -> ("string out"=w322:string, "error out"=w321:errorcluster)  [unwired: 17 in]
        n167 = case shown="Default" w322 {
          selector: w322 -> [_ w324]
          tunnel: w321 -> [w323 w326]
          tunnel: [w323 w325] -> w318
          frame "", "N/A" {
          }
          frame Default {
            n168 = Concatenate Strings("mstsc " ("command line"), w324) -> (w328:string)
            n169 = call <vilib>:"System Exec.vi"("wait until completion? (T)"=FALSE, "error in (no error)"=w326, "command line"=w328) -> ("error out"=w325:errorcluster)  [unwired: 5 in, 3 out]
          }
        }
      }
      event User Event {
        n170 = event-data() -> ("Class"=w333:string)  [unwired: 1 in]
        n171 = call "Z6_Beamline.set GUI Refs.vi"("VI in"=w335, "Class"=w333, "Z6 Beamline GUI Refs"=w332, "PH_BL_Master GUI Refs"=w331, "System Information GUI Refs"=w330, "error in (no error)"=w337) -> ("VI out"=w334:refnum<vi>, "error out"=w336:errorcluster)  [unwired: 12 in]
        n172 = call "PH_Class.set GUI Refs stored Occurence.vi"("i ref in"=w334, "error in (no error)"=w336) -> ("i ref out"=w338:refnum<vi>, "error out"=w339:errorcluster)  [unwired: 16 in]
      }
    }
    "loop counter" <- w147
  }
  "error out" <- w108
  n173 = property on="PCS System Indicator" class="Bool (strict)"("Caption.Text"=w54, "Caption.TextColor"=w53) -> ()  [unwired: 2 in, 2 out]
  n174 = property on="Image Statistician" class="Bool"("Visible"=w52) -> ()  [unwired: 2 in, 2 out]
  n175 = call "PH_Interaction.Super Destroy Me.vi"("i ref out"=w109) -> ()
  n176 = Unregister For Events(event registration refnum=w32) -> ()  [unwired: 1 in, 1 out]
